vi "Write Mode.vi"(8 "Error In":errorcluster, 10 "Mode":T1 items=["Non-Blocking", "Blocking"], 11 "Session In":refnum<class "Session.lvclass">) -> (0 "Error Out":errorcluster, 3 "Sesssion Out":refnum<class "Session.lvclass">)   [LabVIEW 2018, in "Toolkit.lvlib" / "Session.lvclass"]
doc: "Set the communication mode for this session with the remote SSH server."
uses:
  Session.lvclass
  Typedefs/Modes.ctl
  Session.lvclass/Session.ctl
  SSH/SSH.lvclass/SSH.ctl
  Toolkit.lvlib
  SSH/SSH.lvclass
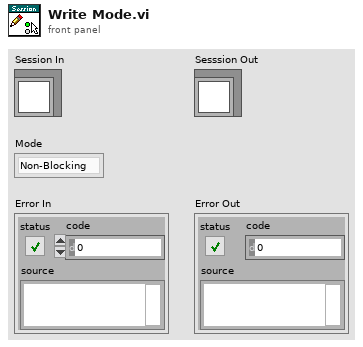
[diagram p1: front panel]
types:
  T1 = typedef "Toolkit.lvlib/Session.lvclass/Modes.ctl" = i32
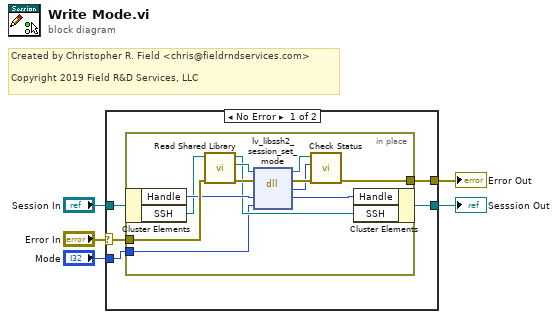
[diagram p0: block diagram]
diagram:
  # "Created by Christopher R. Field <chris@fieldrndservices.com>\n\nCopyright 2019 Field R&D Services, LLC"
  n1 = case shown="No Error" "Error In" {
    selector: "Error In" -> [w9 w24]
    tunnel: [w10 w24] -> w4
    tunnel: "Session In" -> [w8 w23]
    tunnel: [w7 w23] -> w2
    tunnel: "Mode" -> [w6 _]
    frame No Error {
      n2 = in-place {
        in-place-border: [w18] -> w10
        in-place-border: w9 -> [w22]
        in-place-border: w6 -> [w11]
        n3 = in-place-cluster #1(w8) -> ("Handle"=w21:u64, "SSH"=w14:refnum<class "SSH.lvclass">)
        n4 = call "Read Shared Library.vi"("Error In"=w22, "SSH In"=w14) -> ("Error Out"=w15:errorcluster, "lv-libssh2 Shared Library"=w13:path, "SSH Out"=w12:refnum<class "SSH.lvclass">)  [unwired: 7 in]
        n5 = dll-call lib="D:/Users/cfield/Code/Field R&D Services/SSH/LV-LIBSSH2/LabVIEW/trunk/src/Toolkit/Support/lv-libssh2.*" fn="lv_libssh2_session_set_mode"(path in=w13, error in=w15, "session"=w21, "blocking"=w11) -> (path out=w16:path, error out=w19:errorcluster, "status"=w17:i32, "session"=w20:u64)  [unwired: 2 in]
        n6 = call "Check Status.vi"("Error In"=w19, "Status"=w17, "lv-libssh2 Shared Library In"=w16) -> ("Error Out"=w18:errorcluster)  [unwired: 7 in, 1 out]
        n7 = in-place-cluster #1("Handle"=w20, "SSH"=w12) -> (w7:refnum<class "Session.lvclass">)
      }
    }
    frame Error {
    }
  }
  "Sesssion Out" <- w2
  "Error Out" <- w4
